vi "svc_Log View for Spectrum (1Ch).vi"(0 "complex spectrum":T8={"f0"=0.0, "df"=1.0, "complex spectrum"=[]} {"complex spectrum" format="%.2f"; "df" format="%.2f"; "f0" format="%.2f"}, 1 "View":enum16{"Mag-Phase", "Real-Imaginary"}(ring), 9 "spectrum info in":T1={"channel name"="", "description"="", "x-axis units"=0, "spectral info"={"spectrum type"=enum."Power [Magnitude^2]", "linear/dB"=enum."linear", "window"=0, "window size"=0, "FFT size"=0}, "engineering units"=1, "custom label"="", "dB reference [EU]"=0.0, "peak units"=enum."rms", "weighting filter"=0, "spectral density?"=FALSE, "unit label"="", "spectrum skewed?"=FALSE, "complimentary spectrum units"=enum."none"} {"x-axis units" items=["Time (s)"=0, "Frequency-CB (Hz)"=1, "Frequency-CPB (Hz)"=1248, "Frequency-Arbitrary (Hz)"=2357, "Quefrency (s)"=2, "Revolutions (rev)"=3, "Order"=4, "Speed (RPM)"=11, "Speed (rad/s)"=21, "Index"=65535]; "weighting filter" items=["Linear", "A-weighting", "B-weighting", "C-weighting", "ITU-R 468-4", "Dolby", "CCITT", "C-message", "Wb", "Wc", "Wd", "We", "Wf", "Wh", "Wj", "Wk", "Wm", "AES17 20 kHz lowpass", "AES17 40 kHz lowpass", "AES17 20 kHz highpass", "AES17 40 kHz highpass"]; "dB reference [EU]" format="%.2f"; "engineering units" items=["custom..."=0, "V"=1, "A"=21, "C"=30, "pC"=31, "s"=32, "-"=29, "Pa"=2, "N"=20, "g"=3, "m/s^2"=4, "m/s"=5, "m"=6, "mm/s"=12, "mm"=13, "micron/s"=14, "micron"=15, "in/s^2"=7, "in/s"=8, "in"=9, "mil/s"=10, "mil"=11, "rad/s^2"=16, "rad/s"=17, "rad"=18, "deg/s^2"=26, "deg/s"=27, "deg"=28, "RPM"=22, "cycle/s^2"=23, "Hz"=24, "cycle"=25, "strain"=19]; "spectral info"."window" items=["None "=0, "Hanning"=1, "Hamming"=2, "Blackman-Harris"=3, "Exact Blackman"=4, "Blackman"=5, "Flat Top"=6, "4 Term B-Harris "=7, "7 Term B-Harris"=8, "Low Sidelobe"=9, "Force - Exponential"=10, "Gaussian"=62]}, 11 "error in (no error)":errorcluster, 12 "view":T7={"dB On (T)"=TRUE, "unwrap phase (F)"=FALSE, "convert to degree (T)"=TRUE}) -> (3 "unit label [mag or real]":string, 4 "magnitude or real":cluster{"f0":dbl, "df":dbl, dbl[]} {"?" format="%.2f"; "df" format="%.2f"; "f0" format="%.2f"}, 6 "phase or imag":cluster{"f0":dbl, "df":dbl, dbl[]} {"?" format="%.2f"; "df" format="%.2f"; "f0" format="%.2f"}, 10 "spectrum info out":T1={"channel name"="", "description"="", "x-axis units"=0, "spectral info"={"spectrum type"=enum."Power [Magnitude^2]", "linear/dB"=enum."linear", "window"=0, "window size"=0, "FFT size"=0}, "engineering units"=0, "custom label"="", "dB reference [EU]"=0.0, "peak units"=enum."rms", "weighting filter"=0, "spectral density?"=FALSE, "unit label"="", "spectrum skewed?"=FALSE, "complimentary spectrum units"=enum."none"} {"x-axis units" items=["Time (s)"=0, "Frequency-CB (Hz)"=1, "Frequency-CPB (Hz)"=1248, "Frequency-Arbitrary (Hz)"=2357, "Quefrency (s)"=2, "Revolutions (rev)"=3, "Order"=4, "Speed (RPM)"=11, "Speed (rad/s)"=21, "Index"=65535]; "weighting filter" items=["Linear", "A-weighting", "B-weighting", "C-weighting", "ITU-R 468-4", "Dolby", "CCITT", "C-message", "Wb", "Wc", "Wd", "We", "Wf", "Wh", "Wj", "Wk", "Wm", "AES17 20 kHz lowpass", "AES17 40 kHz lowpass", "AES17 20 kHz highpass", "AES17 40 kHz highpass"]; "dB reference [EU]" format="%.2f"; "engineering units" items=["custom..."=0, "V"=1, "A"=21, "C"=30, "pC"=31, "s"=32, "-"=29, "Pa"=2, "N"=20, "g"=3, "m/s^2"=4, "m/s"=5, "m"=6, "mm/s"=12, "mm"=13, "micron/s"=14, "micron"=15, "in/s^2"=7, "in/s"=8, "in"=9, "mil/s"=10, "mil"=11, "rad/s^2"=16, "rad/s"=17, "rad"=18, "deg/s^2"=26, "deg/s"=27, "deg"=28, "RPM"=22, "cycle/s^2"=23, "Hz"=24, "cycle"=25, "strain"=19]; "spectral info"."window" items=["None "=0, "Hanning"=1, "Hamming"=2, "Blackman-Harris"=3, "Exact Blackman"=4, "Blackman"=5, "Flat Top"=6, "4 Term B-Harris "=7, "7 Term B-Harris"=8, "Low Sidelobe"=9, "Force - Exponential"=10, "Gaussian"=62]}, 14 "unit label [phase or imag]":string, 15 "error out":errorcluster)   [LabVIEW 2017]
uses:
  <vilib>/addons/_NISVFA/_Shared subVIs/Controls/svc_Spectrum Info.ctl
  <vilib>/addons/_NISVFA/_Shared subVIs/Controls/svc_X-Axis Units.ctl
  <vilib>/addons/_NISVFA/_Shared subVIs/Controls/svc_Spectrum Type.ctl
  <vilib>/addons/_NISVFA/_Shared subVIs/Controls/svc_Engineering Units Text Ring.ctl
  <vilib>/addons/_NISVFA/_Shared subVIs/Controls/svc_Weighting Filter Text Ring.ctl
  <vilib>/addons/_NISVFA/_Shared subVIs/Controls/svc_Complimentary Spectrum Units.ctl
  <vilib>/addons/_NISVFA/_Shared subVIs/Common/svc_Get Weighting Enum and Labels.vi
  <vilib>/addons/_NISVFA/_Shared subVIs/Common/svc_Unit Label Lexical Class.vi
  <vilib>/addons/_NISVFA/_Shared subVIs/Common/svc_Engineering Units to Unit Label.vi
  <vilib>/addons/_NISVFA/_Shared subVIs/Common/svc_Format Value (DBL).vi
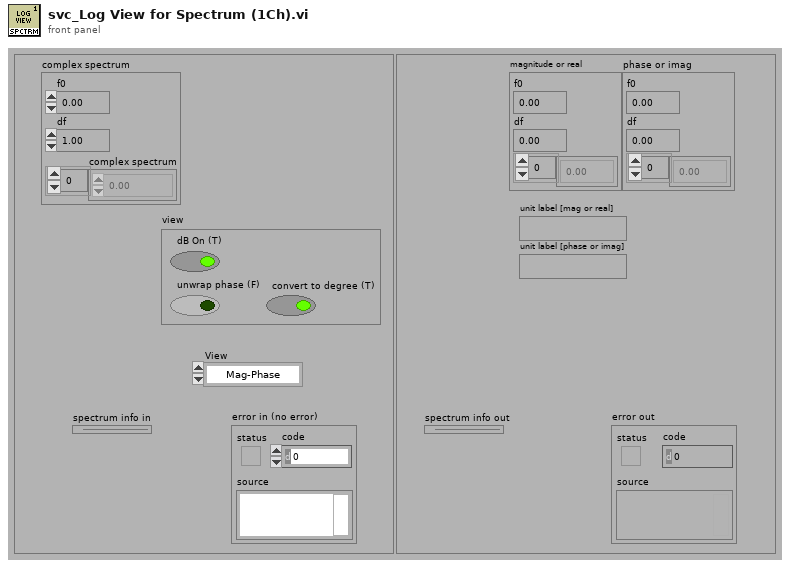
[diagram p1: front panel]
types:
  T1 = typedef "svc_Spectrum Info.ctl" = cluster{"channel name":string, "description":string, "x-axis units":T2, "spectral info":cluster{"spectrum type":T3, "linear/dB":enum16{"linear", "dB"}, "window":u16, "window size":i32, "FFT size":i32}, "engineering units":T4, "custom label":string, "dB reference [EU]":dbl, "peak units":enum16{"rms", "peak", "peak-peak"}, "weighting filter":T5, "spectral density?":bool, "unit label":string, "spectrum skewed?":bool, "complimentary spectrum units":T6}
  T2 = typedef "svc_X-Axis Units.ctl" = u16
  T3 = typedef "svc_Spectrum Type.ctl" = enum16{"FFT Spectrum [complex]", "Amplitude [Magnitude]", "Power [Magnitude^2]", "Cross Spectrum [complex]", "Frequency Response [Complex]"}
  T4 = typedef "svc_Engineering Units Text Ring.ctl" = u16
  T5 = typedef "svc_Weighting Filter Text Ring.ctl" = u16
  T6 = typedef "svc_Complimentary Spectrum Units.ctl" = enum16{"none", "radians", "degrees", "cycles", "imaginary"}
  T7 = cluster{"dB On (T)":bool, "unwrap phase (F)":bool, "convert to degree (T)":bool}
  T8 = cluster{"f0":dbl, "df":dbl, "complex spectrum":cdb[]}
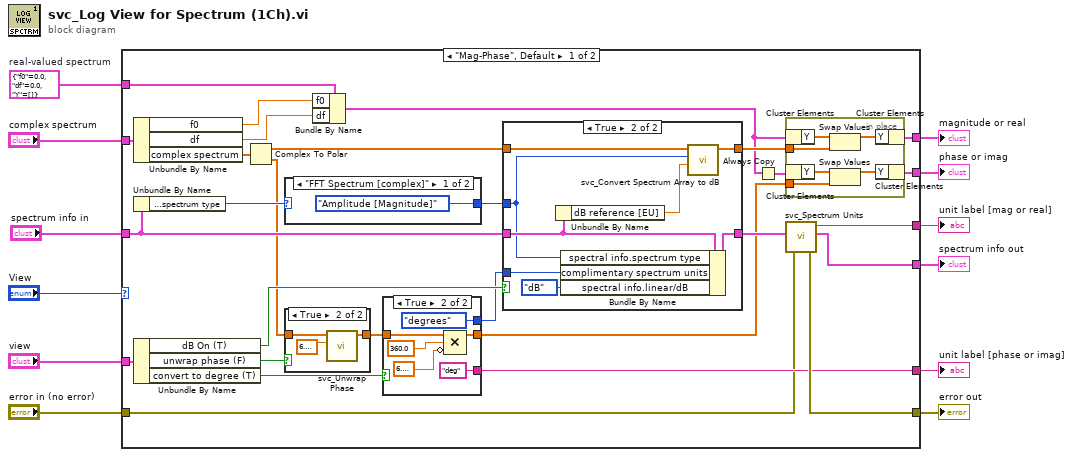
[diagram p0: block diagram]
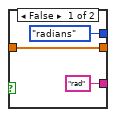
[diagram p4: hidden frame]
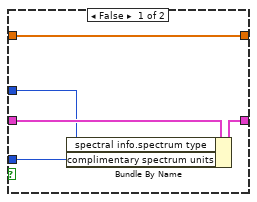
[diagram p5: hidden frame]
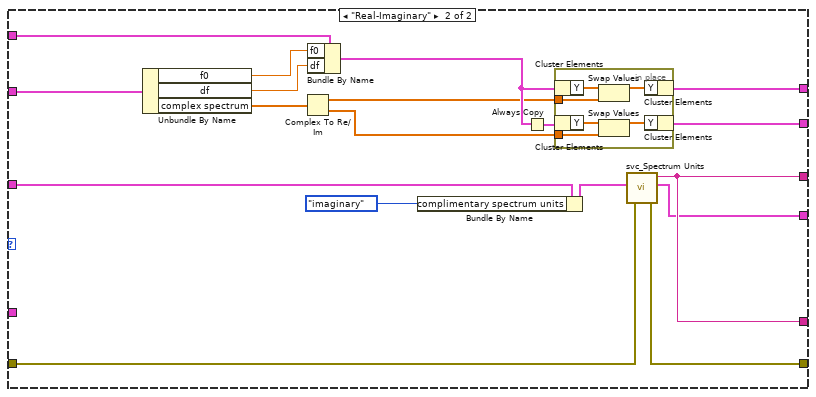
[diagram p6: hidden frame]
diagram:
  w1 = cluster{"f0":dbl, "df":dbl, "Y":dbl[]} {"f0"=0.0, "df"=0.0, "Y"=[]}  # real-valued spectrum
  n1 = case shown="\"Mag-Phase\", Default" "View" {
    tunnel: [w40 w91] -> w10
    tunnel: [w31 w91] -> w9
    tunnel: "complex spectrum" -> [w36 w87]
    tunnel: [w18 w77] -> w7
    tunnel: [w14 w76] -> w8
    tunnel: "error in (no error)" -> [w30 w92]
    tunnel: [w39 w89] -> w6
    tunnel: [w38 w90] -> w4
    tunnel: "view" -> [w37 _]
    tunnel: "spectrum info in" -> [w26 w86]
    tunnel: w1 -> [w13 w75]
    frame "Mag-Phase", Default {
      n2 = Unbundle By Name(w36) -> ("f0"=w21:dbl, "df"=w20:dbl, "complex spectrum"=w35:cdb[])
      n3 = Unbundle By Name(w26) -> ("spectral info.spectrum type"=w25:T3)
      n4 = Unbundle By Name(w37) -> ("dB On (T)"=w28:bool, "unwrap phase (F)"=w33:bool, "convert to degree (T)"=w32:bool)
      n5 = Complex To Polar(r * e^(i*theta)=w35) -> (r=w34:dbl[], theta=w22:dbl[])
      n6 = case shown="\"FFT Spectrum [complex]\"" w25 {
        selector: w25 -> [_ w48]
        tunnel: [svc_Spectrum_Type."Amplitude [Magnitude]" ("spectrum type") w48] -> w27
        frame "FFT Spectrum [complex]" {
        }
        frame Default {
        }
      }
      n7 = case shown="True" w33 {
        tunnel: w22 -> [w49 w52]
        tunnel: [w49 w51] -> w23
        frame False {
        }
        frame True {
          n8 = call <vilib>:"svc_Unwrap Phase.vi"("full cycle (2pi)"=6.283185307179586 ("x"), "phase in"=w52) -> ("phase out"=w51:dbl[])  [unwired: 8 in, 1 out]
        }
      }
      n9 = Bundle By Name(cluster=w13, "f0"=w21, "df"=w20) -> (w17:cluster{"f0":dbl, "df":dbl, "Y":dbl[]})
      n10 = case shown="True" w32 {
        tunnel: [w55 w61] -> w15
        tunnel: w23 -> [w55 w57]
        tunnel: ["rad" ("unit label (phase)") "deg" ("unit label (phase)")] -> w31
        tunnel: [svc_Complimentary_Spectrum_Units."radians" ("complimentary spectrum units") svc_Complimentary_Spectrum_Units."degrees" ("complimentary spectrum units")] -> w24
        frame False {
        }
        frame True {
          n11 = Compound Arithmetic op=MULTIPLY(w57, 360.0 ("x"), invert 6.283185307179586 ("Pi Multiplied By 2")) -> (w61:dbl[])
        }
      }
      n12 = case shown="True" w28 {
        tunnel: w26 -> [w65 w73]
        tunnel: [w64 w74] -> w29
        tunnel: w34 -> [w66 w71]
        tunnel: [w66 w70] -> w19
        tunnel: w27 -> [w63 w69]
        tunnel: w24 -> [w62 w67]
        frame False {
          n13 = Bundle By Name(cluster=w65, "spectral info.spectrum type"=w63, "complimentary spectrum units"=w62) -> (w64:T1)
        }
        frame True {
          n14 = Unbundle By Name(w73) -> ("dB reference [EU]"=w72:dbl)
          n15 = Bundle By Name(cluster=w73, "spectral info.spectrum type"=w69, "complimentary spectrum units"=w67, "spectral info.linear/dB"=enum16{"linear", "dB"}."dB" ("Spectral Info.linear/dB")) -> (w74:T1)
          n16 = call <vilib>:"svc_Convert Spectrum Array to dB.vi"("dB reference"=w72, "spectrum type"=w69, "spectrum"=w71) -> ("spectrum in dB"=w70:dbl[])  [unwired: 8 in]
        }
      }
      n17 = Always Copy(1:w17) -> (0:w16:cluster{"f0":dbl, "df":dbl, "Y":dbl[]})
      n18 = in-place {
        in-place-border: w19 -> [w44]
        in-place-border: w15 -> [w41]
        n19 = in-place-cluster #1(w17) -> ("Y"=w46:dbl[])
        n20 = in-place-cluster #2(w16) -> ("Y"=w43:dbl[])
        n21 = Swap Values(12:w46, 14:w44) -> (1:w45:dbl[])  [unwired: 1 in, 1 out]
        n22 = Swap Values(12:w43, 14:w41) -> (1:w42:dbl[])  [unwired: 1 in, 1 out]
        n23 = in-place-cluster #1("Y"=w45) -> (w18:cluster{"f0":dbl, "df":dbl, "Y":dbl[]})
        n24 = in-place-cluster #2("Y"=w42) -> (w14:cluster{"f0":dbl, "df":dbl, "Y":dbl[]})
      }
      n25 = call <vilib>:"svc_Spectrum Units.vi"("error in (no error)"=w30, "spectrum info in"=w29) -> ("error out"=w39:errorcluster, "spectrum info out"=w38:T1, "unit label"=w40:string)  [unwired: 2 in, 1 out]
    }
    frame "Real-Imaginary" {
      n26 = Unbundle By Name(w87) -> ("f0"=w82:dbl, "df"=w81:dbl, "complex spectrum"=w88:cdb[])
      n27 = Complex To Re/Im(x + iy=w88) -> (x=w79:dbl[], y=w78:dbl[])
      n28 = Bundle By Name(cluster=w75, "f0"=w82, "df"=w81) -> (w80:cluster{"f0":dbl, "df":dbl, "Y":dbl[]})
      n29 = Bundle By Name(cluster=w86, "complimentary spectrum units"=svc_Complimentary_Spectrum_Units."imaginary") -> (w85:T1)
      n30 = Always Copy(1:w80) -> (0:w83:cluster{"f0":dbl, "df":dbl, "Y":dbl[]})
      n31 = in-place {
        in-place-border: w79 -> [w96]
        in-place-border: w78 -> [w93]
        n32 = in-place-cluster #3(w80) -> ("Y"=w98:dbl[])
        n33 = in-place-cluster #4(w83) -> ("Y"=w95:dbl[])
        n34 = Swap Values(12:w98, 14:w96) -> (1:w97:dbl[])  [unwired: 1 in, 1 out]
        n35 = Swap Values(12:w95, 14:w93) -> (1:w94:dbl[])  [unwired: 1 in, 1 out]
        n36 = in-place-cluster #3("Y"=w97) -> (w77:cluster{"f0":dbl, "df":dbl, "Y":dbl[]})
        n37 = in-place-cluster #4("Y"=w94) -> (w76:cluster{"f0":dbl, "df":dbl, "Y":dbl[]})
      }
      n38 = call <vilib>:"svc_Spectrum Units.vi"("error in (no error)"=w92, "spectrum info in"=w85) -> ("error out"=w89:errorcluster, "spectrum info out"=w90:T1, "unit label"=w91:string)  [unwired: 2 in, 1 out]
    }
  }
  "error out" <- w6
  "unit label [mag or real]" <- w10
  "magnitude or real" <- w7
  "unit label [phase or imag]" <- w9
  "phase or imag" <- w8
  "spectrum info out" <- w4
